vi "Recipe downloadv2.vi"() -> ()   [LabVIEW 2014, in "Main Libraryv2.lvlib"]
uses:
  Control/Main Libraryv2.lvlib
panel:
  in  "Recipe Download":u16
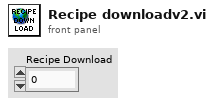
[diagram p1: front panel]
diagram:
